vi "Initialize Event Registrations.vi"(8 "error in (no error)":errorcluster, 11 "Events-References":T1) -> (0 "error out":errorcluster, 3 "Event-Registrations":T2)   [LabVIEW 2018, in "Copy of Actor.lvclass"]
uses:
  Copy of Actor.lvclass
  Event-Registrations.ctl
  Stop.ctl
  Event-References.ctl
  Launched.ctl
  Some Request.ctl
  Some Response.ctl
panel:
  in  "Some":refnum<event-registration>
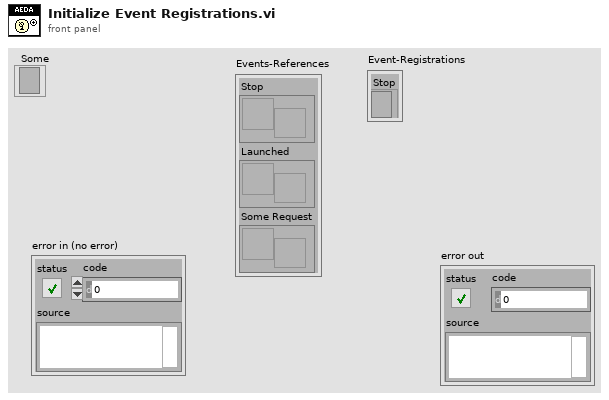
[diagram p1: front panel]
types:
  T1 = typedef "Copy of Actor.lvclass/Event-References.ctl" = cluster{"Stop":refnum<user-event>, "Launched":refnum<user-event>, "Some Request":refnum<user-event>}
  T2 = typedef "Copy of Actor.lvclass/Event-Registrations.ctl" = cluster{"Stop":refnum<event-registration>}
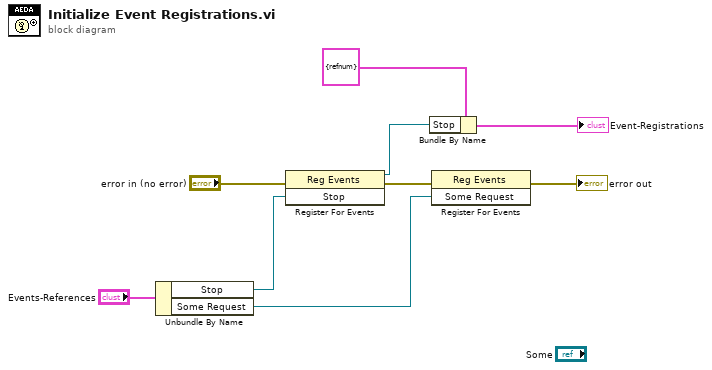
[diagram p0: block diagram]
diagram:
  n1 = Unbundle By Name("Events-References") -> ("Stop"=w6:refnum<user-event>, "Some Request"=w2:refnum<user-event>)
  n2 = register-events(error in="error in (no error)", w6) -> (reference out=w5:refnum<event-registration>, error out=w3:errorcluster)  [unwired: 1 in]
  n3 = Bundle By Name(cluster=T2 {"Stop"=refnum} ("Actor-Event-Registrations"), "Stop"=w5) -> (→"Event-Registrations":T2)
  n4 = register-events(error in=w3, w2) -> (error out=→"error out":errorcluster)  [unwired: 1 in, 1 out]
